vi "Number of Tabs - Maximum--Const.vi"() -> (3 "Maximum Tabs":i32)   [LabVIEW 2017, in "DTacq Plot Display Library.lvlib"]
uses:
  DTacq Plot Display Library.lvlib
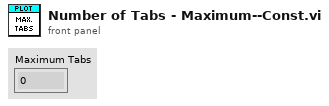
[diagram p1: front panel]
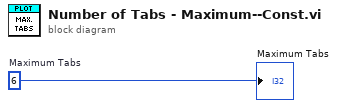
[diagram p0: block diagram]
diagram:
  w1 = 6  # Maximum Tabs
  "Maximum Tabs" <- w1
